vi "Hide Animated Busy Icon with Message.vi"(4 "Animated Busy Icon Control Name (Animated Busy Icon)":string="Animated Busy Icon", 5 "Already active? (F)":bool, 6 "Message Control Name (Message)":string="Message", 7 "Message":string, 9 "Error In":errorcluster, 11 "Target VI reference":refnum<vi>) -> (1 "Error Out":errorcluster)   [LabVIEW 2021, in "GUI.lvlib"]
doc: "This VI passes error in through and ignores it."
uses:
  GUI/GUI.lvlib
  Error/Error.lvlib
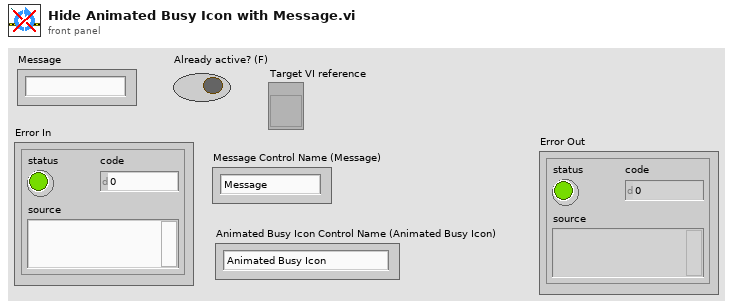
[diagram p1: front panel]
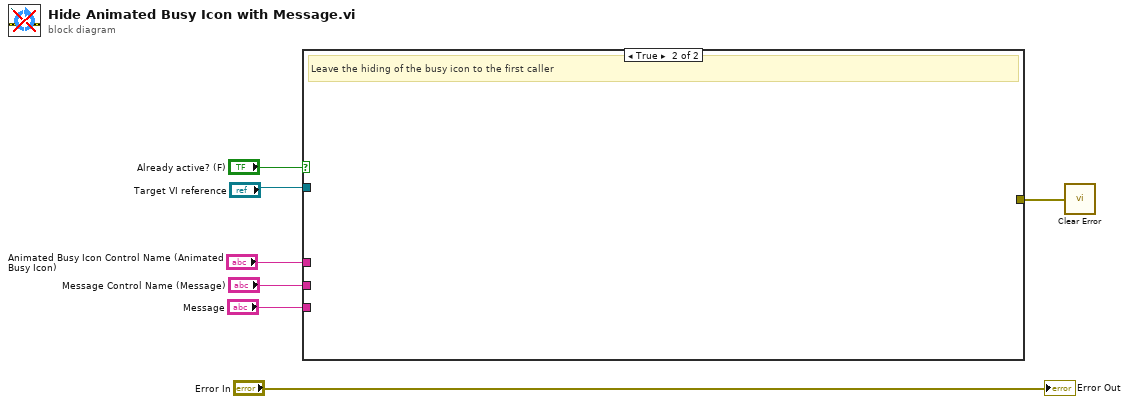
[diagram p0: block diagram]
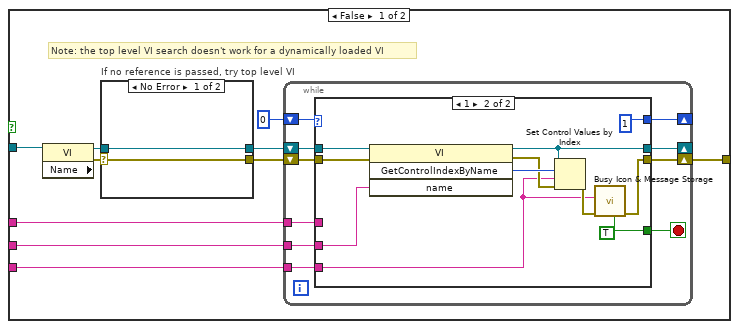
[diagram p2: hidden frame]
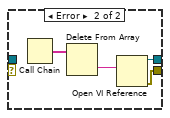
[diagram p3: hidden frame]
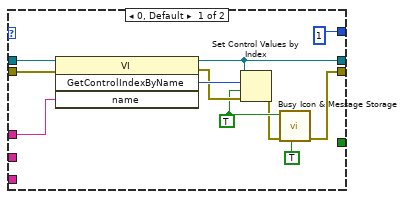
[diagram p4: hidden frame]
diagram:
  n1 = case shown="True" "Already active? (F)" {
    tunnel: [w17 _] -> w1
    tunnel: "Message Control Name (Message)" -> [w15 _]
    tunnel: "Animated Busy Icon Control Name (Animated Busy Icon)" -> [w14 _]
    tunnel: "Message" -> [w13 _]
    tunnel: "Target VI reference" -> [w10 _]
    frame False {
      # "Note: the top level VI search doesn't work for a dynamically loaded VI"
      n2 = property class="VI" props=["Name"](reference=w10) -> (reference out=w9:refnum<vi>, error out=w8:errorcluster)  [unwired: 1 in, 1 out]
      n3 = case "If no reference is passed, try top level VI" shown="No Error" w8 {
        selector: w8 -> [w18 _]
        tunnel: [w18 w23] -> w11
        tunnel: [w19 w22] -> w12
        tunnel: w9 -> [w19 _]
        frame No Error {
        }
        frame Error {
          n4 = Call Chain() -> (call chain=w20:string[])
          n5 = Delete From Array(array=w20) -> (deleted portion=w21:string)  [unwired: 2 in, 1 out]
          n6 = Open VI Reference(vi path=w21) -> (vi reference=w22:refnum<vi>, error out=w23:errorcluster)  [unwired: 5 in]
        }
      }
      n7 = while {
        shift-right: [w30] -> w17
        shift-left: w11 -> [w33]
        shift-right: [w31] -> _
        shift-left: w12 -> [w32]
        shift-right: [w28] -> _
        shift-left: 0 -> [w29]
        tunnel: w15 -> [w26]
        tunnel: w14 -> [w25]
        tunnel: w13 -> [w24]
        stop <- w27 stop-if-true
        n8 = case shown="1" w29 {
          tunnel: w33 -> [w42 w53]
          tunnel: w32 -> [w41 w52]
          tunnel: [w40 w51] -> w31
          tunnel: [w34 w47] -> w30
          tunnel: [1 1] -> w28
          tunnel: [_ w45] -> w27
          tunnel: w26 -> [_ w49]
          tunnel: w25 -> [w38 _]
          tunnel: w24 -> [_ w46]
          frame 0, Default {
            w36 = TRUE ("Visible")
            n9 = invoke class="VI" method="GetControlIndexByName"(reference=w41, error in=w42, "name"=w38) -> (reference out=w40:refnum<vi>, error out=w43:errorcluster, "GetControlIndexByName"=w44:i32)  [unwired: 1 in, 1 out]
            n10 = Set Control Values by Index(0:w40, 1:w44, 2:w36, 3:w43) -> (11:w35:errorcluster)
            n11 = call "Busy Icon & Message Storage.vi"("Get(F)/Set Busy Icon"=TRUE, "Error In"=w35, "Busy Icon Status (F = busy)"=w36) -> ("Error Out"=w34:errorcluster)  [unwired: 6 in, 2 out]
          }
          frame 1 {
            w45 = TRUE
            n12 = invoke class="VI" method="GetControlIndexByName"(reference=w52, error in=w53, "name"=w49) -> (reference out=w51:refnum<vi>, error out=w54:errorcluster, "GetControlIndexByName"=w55:i32)  [unwired: 1 in, 1 out]
            n13 = Set Control Values by Index(0:w51, 1:w55, 2:w46, 3:w54) -> (11:w48:errorcluster)
            n14 = call "Busy Icon & Message Storage.vi"("Get(F)/Set Message"=w45, "Error In"=w48, "Message String"=w46) -> ("Error Out"=w47:errorcluster)  [unwired: 6 in, 2 out]
          }
        }
      }
    }
    frame True {
      # "Leave the hiding of the busy icon to the first caller"
    }
  }
  n15 = call "Clear Error.vi"("Error In"=w1) -> ()  [unwired: 8 in, 1 out]
  "Error Out" <- "Error In"
